vi "Vision Processing.vi"(4 "error in (no error)":errorcluster, 7 "Image Size":T1=enum."320x240") -> ()   [LabVIEW 2016]
doc: "This VI runs in parallel to other tasks. It gets images from the camera, processes them for color or shape and use that information to affect robot behavior."
uses:
  <vilib>/Rock Robotics/WPI/Camera/WPI_CameraImageSize.ctl
  <vilib>/Rock Robotics/WPI/Camera/WPI_CameraWhite Balance Values.ctl
  <vilib>/Rock Robotics/WPI/Camera/WPI_CameraExposure Values.ctl
  <vilib>/Rock Robotics/WPI/Camera/WPI_CameraFrameRate.ctl
  Robot Global Data.vi
panel:
  in  "Image Size 2":T1=enum."320x240"
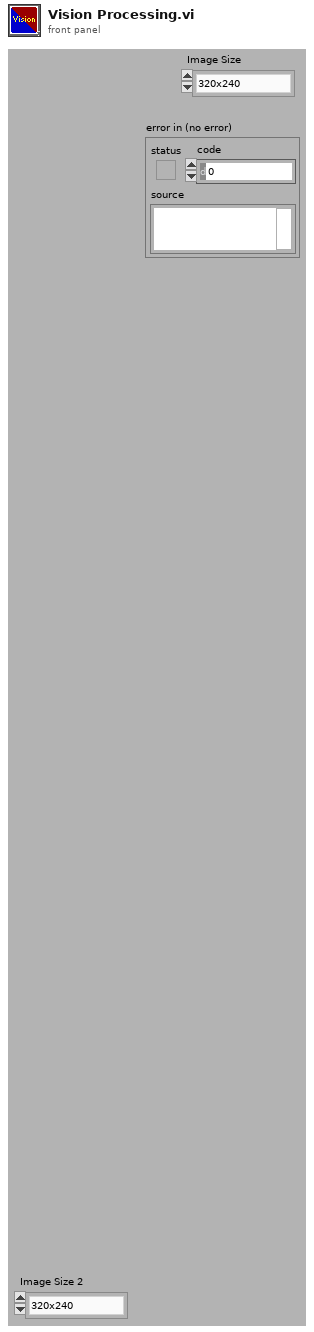
[diagram p1: front panel]
types:
  T1 = typedef "WPI_CameraImageSize.ctl" = enum16{"640x480", "320x240", "160x120", "Custom"}
  T2 = typedef "WPI_CameraFrameRate.ctl" = u32
  T3 = typedef "WPI_CameraExposure Values.ctl" = enum16{"Auto", "Flicker-free 50 Hz", "Flicker-free 60 Hz", "Hold current", "Custom"}
  T4 = typedef "WPI_CameraWhite Balance Values.ctl" = enum16{"Auto", "Fixed indoor", "Fixed outdoor 1", "Fixed outdoor 2", "Fixed fluorescent 1", "Fixed fluorescent 2", "Hold current", "Custom"}
  T5 = typedef "Image Type" = u32
  T6 = typedef "WPI_CameraDevRef.ctl" = cluster{"Camera Address":string, "CameraStatus":errorcluster}
  T7 = typedef "IMAQ Image.ctl" = refnum<image>
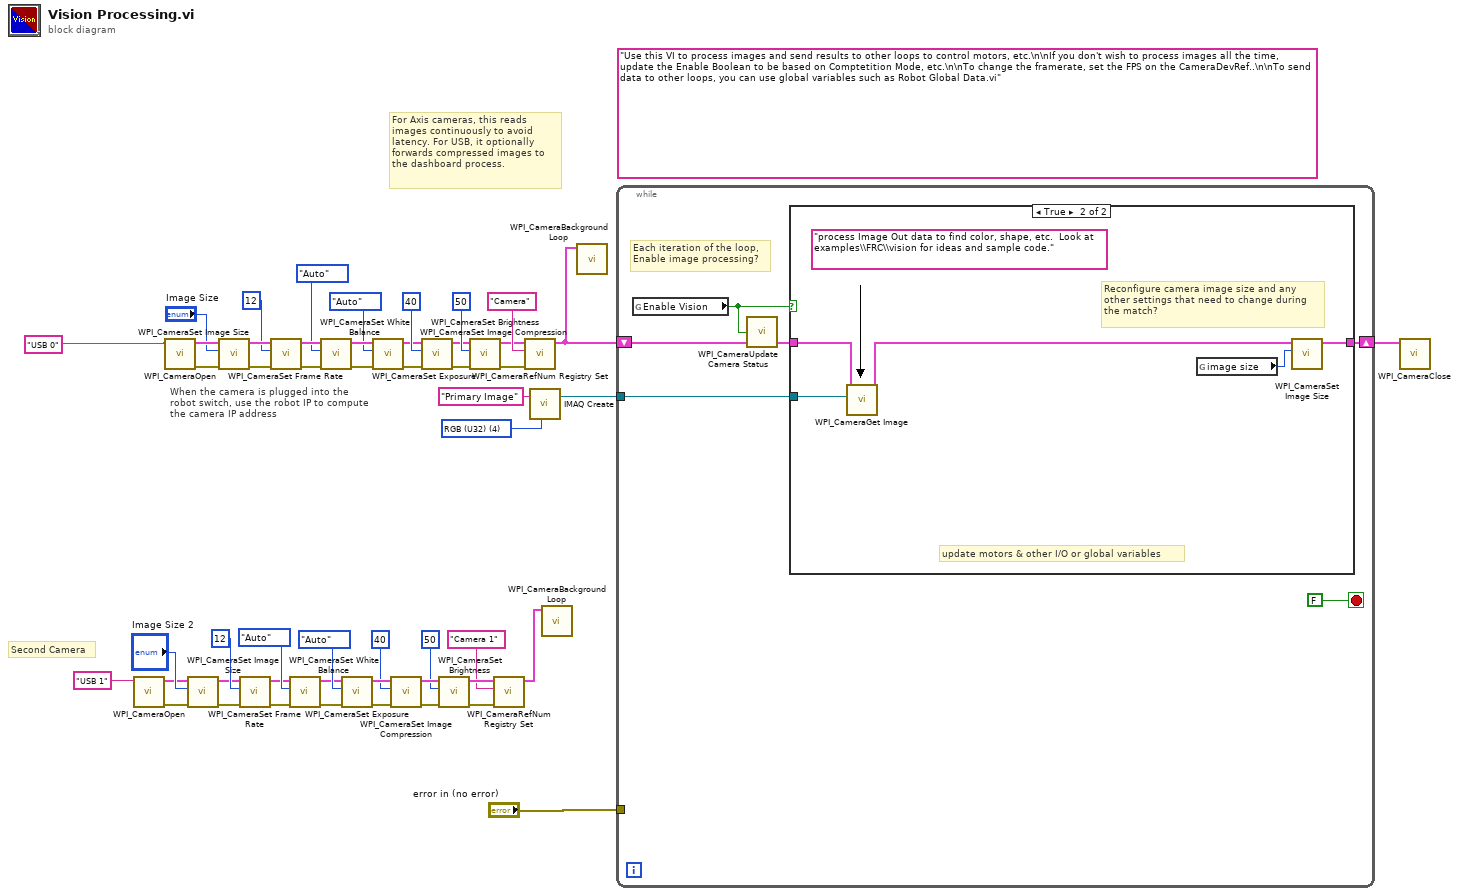
[diagram p0: block diagram]
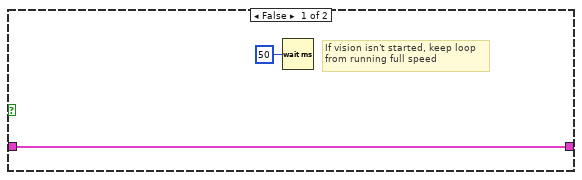
[diagram p2: hidden frame]
diagram:
  (unwired) "Use this VI to process images and send results to other loops to control motors, etc.\n\nIf you don't wish to process images all the time, update the Enable Boolean to be based on Comptetition Mode, etc.\n\nTo change the framerate, set the FPS on the CameraDevRef..\n\nTo send data to other loops, you can use global variables such as Robot Global Data.vi"
  w51 = T5 4 items=["Grayscale (U8)", "Grayscale (I16)", "Grayscale (SGL)", "Complex (CSG)", "RGB (U32)", "HSL (U32)", "RGB (U64)"] ("Image Type")
  # "Second Camera"
  # "When the camera is plugged into the\nrobot switch, use the robot IP to compute\nthe camera IP address"
  # "For Axis cameras, this reads\nimages continuously to avoid\nlatency. For USB, it optionally\nforwards compressed images to\nthe dashboard process."
  n1 = call <vilib>:"WPI_CameraOpen.vi"("Camera Address"="USB 1" ("format string")) -> ("error out"=w12:errorcluster, "CameraDevRef"=w11:T6)  [unwired: 1 in, 8 out]
  n2 = call <vilib>:"WPI_CameraOpen.vi"("Camera Address"="USB 0" ("format string")) -> ("error out"=w39:errorcluster, "CameraDevRef"=w40:T6)  [unwired: 1 in, 8 out]
  n3 = call <vilib>:"WPI_CameraSet Image Size.vi"("error in (no error)"=w12, "Image Size"="Image Size 2", "CameraDevRef"=w11) -> ("error out"=w13:errorcluster, "CameraDevRef Out"=w10:T6)  [unwired: 1 in, 6 out]
  n4 = call <vilib>:"WPI_CameraSet Image Size.vi"("error in (no error)"=w39, "Image Size"="Image Size", "CameraDevRef"=w40) -> ("error out"=w38:errorcluster, "CameraDevRef Out"=w41:T6)  [unwired: 1 in, 6 out]
  n5 = call <vilib>:"WPI_CameraSet Frame Rate.vi"("error in (no error)"=w13, "Frame Rate (fps)"=T2 12, "CameraDevRef"=w10) -> ("error out"=w14:errorcluster, "CameraDevRef Out"=w8:T6)  [unwired: 7 out]
  n6 = call <vilib>:"WPI_CameraSet Frame Rate.vi"("error in (no error)"=w38, "Frame Rate (fps)"=T2 12, "CameraDevRef"=w41) -> ("error out"=w37:errorcluster, "CameraDevRef Out"=w43:T6)  [unwired: 7 out]
  n7 = call <vilib>:"WPI_CameraSet White Balance.vi"("error in (no error)"=w14, "White Balance"=WPI_CameraWhite_Balance_Values."Auto", "CameraDevRef"=w8) -> ("error out"=w15:errorcluster, "CameraDevRef Out"=w9:T6)  [unwired: 1 in, 6 out]
  n8 = call <vilib>:"WPI_CameraSet White Balance.vi"("error in (no error)"=w37, "White Balance"=WPI_CameraWhite_Balance_Values."Auto", "CameraDevRef"=w43) -> ("error out"=w36:errorcluster, "CameraDevRef Out"=w42:T6)  [unwired: 1 in, 6 out]
  n9 = call <vilib>:"WPI_CameraSet Exposure.vi"("error in (no error)"=w15, "Exposure"=WPI_CameraExposure_Values."Auto", "CameraDevRef"=w9) -> ("error out"=w16:errorcluster, "CameraDevRef Out"=w6:T6)  [unwired: 1 in, 6 out]
  n10 = call <vilib>:"WPI_CameraSet Exposure.vi"("error in (no error)"=w36, "Exposure"=WPI_CameraExposure_Values."Auto", "CameraDevRef"=w42) -> ("error out"=w35:errorcluster, "CameraDevRef Out"=w45:T6)  [unwired: 1 in, 6 out]
  n11 = call <vilib>:"WPI_CameraSet Image Compression.vi"("error in (no error)"=w16, "Compression"=40, "CameraDevRef"=w6) -> ("error out"=w17:errorcluster, "CameraDevRef Out"=w7:T6)  [unwired: 7 out]
  n12 = call <vilib>:"WPI_CameraSet Image Compression.vi"("error in (no error)"=w35, "Compression"=40, "CameraDevRef"=w45) -> ("error out"=w34:errorcluster, "CameraDevRef Out"=w44:T6)  [unwired: 7 out]
  n13 = call <vilib>:"WPI_CameraSet Brightness.vi"("error in (no error)"=w17, "Brightness"=50, "CameraDevRef"=w7) -> ("error out"=w19:errorcluster, "CameraDevRef Out"=w18:T6)  [unwired: 7 out]
  n14 = call <vilib>:"WPI_CameraSet Brightness.vi"("error in (no error)"=w34, "Brightness"=50, "CameraDevRef"=w44) -> ("error out"=w32:errorcluster, "CameraDevRef Out"=w33:T6)  [unwired: 7 out]
  n15 = call <vilib>:"WPI_CameraRefNum Registry Set.vi"("error in (no error)"=w19, "refnum name"="Camera 1", "CameraDevRef"=w18) -> ("CameraDevRef"=w23:T6)  [unwired: 1 in, 7 out]
  n16 = call <vilib>:"WPI_CameraRefNum Registry Set.vi"("error in (no error)"=w32, "refnum name"="Camera", "CameraDevRef"=w33) -> ("CameraDevRef"=w28:T6)  [unwired: 1 in, 7 out]
  n17 = call "IMAQ Create"("Image Name"="Primary Image", "Image Type"=w51) -> ("New Image"=w49:T7)  [unwired: 2 in, 2 out]
  n18 = call <vilib>:"WPI_CameraBackground Loop.vi"("CameraDevRef"=w23) -> ()  [unwired: 11 in]
  n19 = call <vilib>:"WPI_CameraBackground Loop.vi"("CameraDevRef"=w28) -> ()  [unwired: 11 in]
  n20 = while {
    shift-right: [w56] -> w26
    shift-left: w28 -> [w54]
    tunnel: w49 -> [w55]
    tunnel: "error in (no error)" -> [_]
    stop <- FALSE stop-if-true
    # "Each iteration of the loop,\nEnable image processing?"
    n21 = global read "Robot Global Data.vi" "Enable Vision"() -> (w52:bool)
    n22 = call <vilib>:"WPI_CameraUpdate Camera Status.vi"("CameraDevRef In"=w54, "Enable Vision"=w52) -> ("CameraDevRef Out"=w53:T6)  [unwired: 3 in]
    n23 = case shown="True" w52 {
      tunnel: w55 -> [_ w63]
      tunnel: [w59 w64] -> w56
      tunnel: w53 -> [w59 w61]
      frame False {
        # "If vision isn't started, keep loop\nfrom running full speed"
        n24 = Wait (ms)(milliseconds to wait=u32 50) -> ()  [unwired: 1 out]
      }
      frame True {
        (unwired) "process Image Out data to find color, shape, etc.  Look at examples\\FRC\\vision for ideas and sample code."
        # "update motors & other I/O or global variables"
        # "Reconfigure camera image size and any\nother settings that need to change during\nthe match?"
        n25 = call <vilib>:"WPI_CameraGet Image.vi"("Image"=w63, "CameraDevRef"=w61) -> ("CameraDevRef Out"=w60:T6)  [unwired: 1 in, 8 out]
        n26 = global read "Robot Global Data.vi" "image size"() -> (w62:T1)
        n27 = call <vilib>:"WPI_CameraSet Image Size.vi"("Image Size"=w62, "CameraDevRef"=w60) -> ("CameraDevRef Out"=w64:T6)  [unwired: 2 in, 7 out]
      }
    }
  }
  n28 = call <vilib>:"WPI_CameraClose.vi"("CameraDevRef"=w26) -> ()  [unwired: 1 in, 10 out]
